vi "Create.vi"(8 "error in (no error)":errorcluster, 10 "reference":refnum<vi>, 11 "subpanel (abstract) in":refnum<class "subpanel (abstract).lvclass">) -> (0 "error out":errorcluster, 2 "data value reference":refnum<data-value>, 3 "subpanel (abstract) out":refnum<class "subpanel (abstract).lvclass">)   [LabVIEW 2023, in "GUI.lvlib" / "subpanel (abstract).lvclass"]
uses:
  subpanel (abstract).lvclass
  subpanel (abstract).lvclass/subpanel (abstract).ctl
  plugins/subPanelHorizontal.vi
  plugins/subPanelVertical.vi
  GUI.lvlib
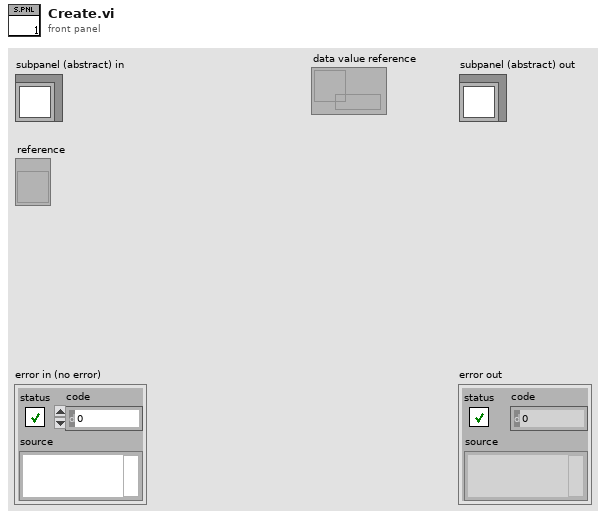
[diagram p1: front panel]
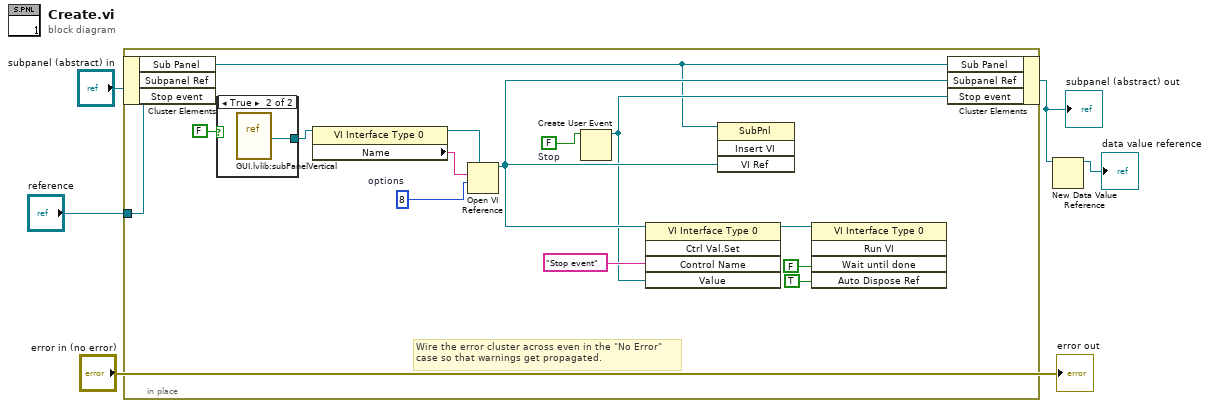
[diagram p0: block diagram]
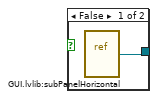
[diagram p2: hidden frame]
diagram:
  n1 = in-place {
    in-place-border: "reference" -> [w6]
    w13 = FALSE  # Stop
    w14 = 8  # options
    # "Wire the error cluster across even in the \"No Error\"\ncase so that warnings get propagated."
    n2 = in-place-cluster #1("subpanel (abstract) in") -> ()  [unwired: 3 out]
    n3 = case shown="True" FALSE {
      tunnel: [w19 w20] -> w7
      frame False {
        n4 = vi-ref "GUI.lvlib:subPanelHorizontal.vi"() -> (w19:refnum<vi>)
      }
      frame True {
        n5 = vi-ref "GUI.lvlib:subPanelVertical.vi"() -> (w20:refnum<vi>)
      }
    }
    n6 = property class="VI Interface Type 0"(reference=w7) -> (reference out=w15:refnum<vi>, "Name"=w16:string)  [unwired: 1 in, 1 out]
    n7 = Open VI Reference(type specifier VI Refnum (for type only)=w15, vi path=w16, options=w14) -> (vi reference=w10:refnum<vi>)  [unwired: 3 in, 1 out]
    n8 = Create User Event(user event datatype=w13) -> (user event=w9:refnum<user-event>)  [unwired: 1 in, 1 out]
    n9 = invoke class="VI Interface Type 0" method="Ctrl Val.Set"(reference=w10, "Control Name"="Stop event", "Value"=w9) -> (reference out=w11:refnum<vi>)  [unwired: 2 in, 4 out]
    n10 = invoke on="Invoke Node" class="SubPnl" method="Insert VI"(reference=w6, "VI Ref"=w10) -> ()  [unwired: 2 in, 4 out]
    n11 = invoke class="VI Interface Type 0" method="Run VI"(reference=w11, "Wait until done"=FALSE ("Wait Until Done"), "Auto Dispose Ref"=TRUE ("Auto Dispose Reference")) -> ()  [unwired: 2 in, 5 out]
    n12 = in-place-cluster #1("Sub Panel"=w6, "Subpanel Ref"=w10, "Stop event"=w9) -> (w3:refnum<class "subpanel (abstract).lvclass">)
  }
  "subpanel (abstract) out" <- w3
  n13 = New Data Value Reference(data value=w3) -> (data value reference=→"data value reference":refnum<data-value>)  [unwired: 1 in, 1 out]
  "error out" <- "error in (no error)"
